vi "Init Log.vi"(8 "error in (no error)":errorcluster, 11 "S4GUI in":refnum<class "S4GUI.lvclass">) -> (0 "error out":errorcluster, 3 "S4GUI out":refnum<class "S4GUI.lvclass">)   [LabVIEW 2018, in "S4GUI.lvclass"]
uses:
  S4GUI.lvclass
  S4GUI.lvclass/S4GUI.ctl
  Log/Log.lvclass
  Acquisition/Acquisition.lvclass
  Instrument/Instrument.lvclass
  TCS/TCS.lvclass
  SyncBox/Sync Box.lvclass
  TelFocus/TelFocus.lvclass
  Comm/Stream/Stream.lvclass
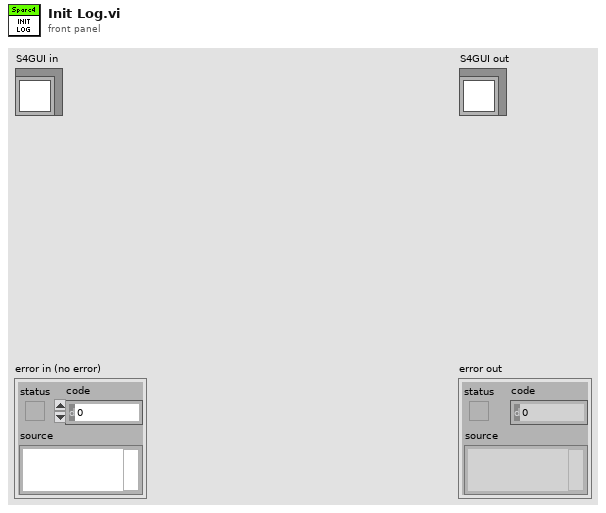
[diagram p1: front panel]
types:
  T1 = enum16{"open", "replace", "create", "open or create", "replace or create", "replace or create with confirmation"}
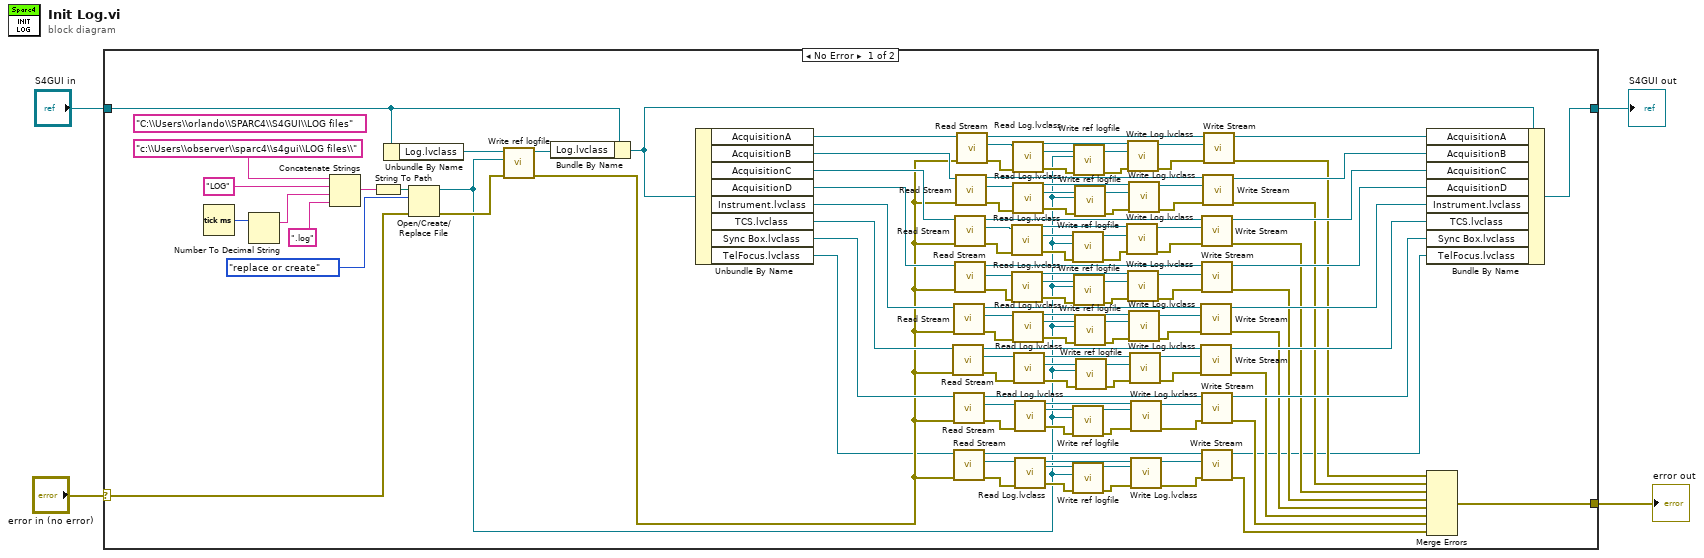
[diagram p0: block diagram]
diagram:
  n1 = case shown="No Error" "error in (no error)" {
    selector: "error in (no error)" -> [w123 w128]
    tunnel: [w98 w128] -> w3
    tunnel: [w120 w127] -> w1
    tunnel: "S4GUI in" -> [w24 w127]
    frame No Error {
      (unwired) "C:\\Users\\orlando\\SPARC4\\S4GUI\\LOG files"
      n2 = Tick Count (ms)() -> (millisecond timer value=w95:u32)
      n3 = Number To Decimal String(number=w95) -> (decimal integer string=w94:string)  [unwired: 1 in]
      n4 = Concatenate Strings("c:\\Users\\observer\\sparc4\\s4gui\\LOG files\\" ("string"), "LOG" ("string"), w94, ".log" ("string")) -> (w124:string)
      n5 = String To Path(string=w124) -> (path=w125:path)
      n6 = Unbundle By Name(w24) -> ("Log.lvclass"=w22:refnum<class "Log.lvclass">)
      n7 = Open/Create/Replace File(file path (use dialog)=w125, error in=w123, operation (0:open)=T1."replace or create") -> (refnum out=w6:refnum<file>, error out=w23:errorcluster)  [unwired: 3 in, 1 out]
      n8 = call-dynamic "Write ref logfile.vi"("error in (no error)"=w23, "ref logfile"=w6, "Log in"=w22) -> ("error out"=w13:errorcluster, "Log out"=w21:refnum<class "Log.lvclass">)  [unwired: 7 in]
      n9 = Bundle By Name(cluster=w24, "Log.lvclass"=w21) -> (w121:refnum<class "S4GUI.lvclass">)
      n10 = Unbundle By Name(w121) -> ("AcquisitionA"=w119:refnum<class "Acquisition.lvclass">, "AcquisitionB"=w118:refnum<class "Acquisition.lvclass">, "AcquisitionC"=w117:refnum<class "Acquisition.lvclass">, "AcquisitionD"=w116:refnum<class "Acquisition.lvclass">, "Instrument.lvclass"=w115:refnum<class "Instrument.lvclass">, "TCS.lvclass"=w114:refnum<class "TCS.lvclass">, "Sync Box.lvclass"=w113:refnum<class "Sync Box.lvclass">, "TelFocus.lvclass"=w12:refnum<class "TelFocus.lvclass">)
      n11 = call-dynamic "Read Stream.vi"("error in (no error)"=w13, "Server in"=w114) -> ("error out"=w30:errorcluster, "Stream.lvclass"=w31:refnum<class "Stream.lvclass">, "Server out"=w34:refnum<class "TCS.lvclass">)  [unwired: 7 in]
      n12 = call-dynamic "Read Stream.vi"("error in (no error)"=w13, "Server in"=w115) -> ("error out"=w46:errorcluster, "Stream.lvclass"=w48:refnum<class "Stream.lvclass">, "Server out"=w49:refnum<class "Instrument.lvclass">)  [unwired: 7 in]
      n13 = call-dynamic "Read Stream.vi"("error in (no error)"=w13, "Server in"=w113) -> ("error out"=w27:errorcluster, "Stream.lvclass"=w28:refnum<class "Stream.lvclass">, "Server out"=w29:refnum<class "Sync Box.lvclass">)  [unwired: 7 in]
      n14 = call-dynamic "Read Stream.vi"("error in (no error)"=w13, "Server in"=w12) -> ("error out"=w15:errorcluster, "Stream.lvclass"=w16:refnum<class "Stream.lvclass">, "Server out"=w11:refnum<class "TelFocus.lvclass">)  [unwired: 7 in]
      n15 = call-dynamic "Read Stream.vi"("error in (no error)"=w13, "Server in"=w117) -> ("error out"=w61:errorcluster, "Stream.lvclass"=w63:refnum<class "Stream.lvclass">, "Server out"=w64:refnum<class "Acquisition.lvclass">)  [unwired: 7 in]
      n16 = call-dynamic "Read Stream.vi"("error in (no error)"=w13, "Server in"=w116) -> ("error out"=w56:errorcluster, "Stream.lvclass"=w55:refnum<class "Stream.lvclass">, "Server out"=w59:refnum<class "Acquisition.lvclass">)  [unwired: 7 in]
      n17 = call-dynamic "Read Stream.vi"("error in (no error)"=w13, "Server in"=w118) -> ("error out"=w79:errorcluster, "Stream.lvclass"=w78:refnum<class "Stream.lvclass">, "Server out"=w76:refnum<class "Acquisition.lvclass">)  [unwired: 7 in]
      n18 = call-dynamic "Read Stream.vi"("error in (no error)"=w13, "Server in"=w119) -> ("error out"=w89:errorcluster, "Stream.lvclass"=w93:refnum<class "Stream.lvclass">, "Server out"=w122:refnum<class "Acquisition.lvclass">)  [unwired: 7 in]
      n19 = call-dynamic "Read Log.lvclass.vi"("error in (no error)"=w61, "Comm in"=w63) -> ("error out"=w71:errorcluster, "Log.lvclass"=w74:refnum<class "Log.lvclass">, "Comm out"=w73:refnum<class "Stream.lvclass">)  [unwired: 7 in]
      n20 = call-dynamic "Read Log.lvclass.vi"("error in (no error)"=w56, "Comm in"=w55) -> ("error out"=w66:errorcluster, "Log.lvclass"=w69:refnum<class "Log.lvclass">, "Comm out"=w68:refnum<class "Stream.lvclass">)  [unwired: 7 in]
      n21 = call-dynamic "Read Log.lvclass.vi"("error in (no error)"=w89, "Comm in"=w93) -> ("error out"=w88:errorcluster, "Log.lvclass"=w92:refnum<class "Log.lvclass">, "Comm out"=w91:refnum<class "Stream.lvclass">)  [unwired: 7 in]
      n22 = call-dynamic "Read Log.lvclass.vi"("error in (no error)"=w79, "Comm in"=w78) -> ("error out"=w81:errorcluster, "Log.lvclass"=w84:refnum<class "Log.lvclass">, "Comm out"=w83:refnum<class "Stream.lvclass">)  [unwired: 7 in]
      n23 = call-dynamic "Read Log.lvclass.vi"("error in (no error)"=w46, "Comm in"=w48) -> ("error out"=w51:errorcluster, "Log.lvclass"=w54:refnum<class "Log.lvclass">, "Comm out"=w53:refnum<class "Stream.lvclass">)  [unwired: 7 in]
      n24 = call-dynamic "Read Log.lvclass.vi"("error in (no error)"=w30, "Comm in"=w31) -> ("error out"=w41:errorcluster, "Log.lvclass"=w44:refnum<class "Log.lvclass">, "Comm out"=w43:refnum<class "Stream.lvclass">)  [unwired: 7 in]
      n25 = call-dynamic "Read Log.lvclass.vi"("error in (no error)"=w27, "Comm in"=w28) -> ("error out"=w36:errorcluster, "Log.lvclass"=w39:refnum<class "Log.lvclass">, "Comm out"=w38:refnum<class "Stream.lvclass">)  [unwired: 7 in]
      n26 = call-dynamic "Read Log.lvclass.vi"("error in (no error)"=w15, "Comm in"=w16) -> ("error out"=w18:errorcluster, "Log.lvclass"=w20:refnum<class "Log.lvclass">, "Comm out"=w9:refnum<class "Stream.lvclass">)  [unwired: 7 in]
      n27 = call-dynamic "Write ref logfile.vi"("error in (no error)"=w71, "ref logfile"=w6, "Log in"=w74) -> ("error out"=w70:errorcluster, "Log out"=w72:refnum<class "Log.lvclass">)  [unwired: 7 in]
      n28 = call-dynamic "Write ref logfile.vi"("error in (no error)"=w36, "ref logfile"=w6, "Log in"=w39) -> ("error out"=w35:errorcluster, "Log out"=w37:refnum<class "Log.lvclass">)  [unwired: 7 in]
      n29 = call-dynamic "Write ref logfile.vi"("error in (no error)"=w18, "ref logfile"=w6, "Log in"=w20) -> ("error out"=w17:errorcluster, "Log out"=w19:refnum<class "Log.lvclass">)  [unwired: 7 in]
      n30 = call-dynamic "Write ref logfile.vi"("error in (no error)"=w88, "ref logfile"=w6, "Log in"=w92) -> ("error out"=w87:errorcluster, "Log out"=w90:refnum<class "Log.lvclass">)  [unwired: 7 in]
      n31 = call-dynamic "Write ref logfile.vi"("error in (no error)"=w66, "ref logfile"=w6, "Log in"=w69) -> ("error out"=w65:errorcluster, "Log out"=w67:refnum<class "Log.lvclass">)  [unwired: 7 in]
      n32 = call-dynamic "Write ref logfile.vi"("error in (no error)"=w81, "ref logfile"=w6, "Log in"=w84) -> ("error out"=w80:errorcluster, "Log out"=w82:refnum<class "Log.lvclass">)  [unwired: 7 in]
      n33 = call-dynamic "Write ref logfile.vi"("error in (no error)"=w51, "ref logfile"=w6, "Log in"=w54) -> ("error out"=w50:errorcluster, "Log out"=w52:refnum<class "Log.lvclass">)  [unwired: 7 in]
      n34 = call-dynamic "Write ref logfile.vi"("error in (no error)"=w41, "ref logfile"=w6, "Log in"=w44) -> ("error out"=w40:errorcluster, "Log out"=w42:refnum<class "Log.lvclass">)  [unwired: 7 in]
      n35 = call-dynamic "Write Log.lvclass.vi"("error in (no error)"=w70, "Log.lvclass"=w72, "Comm in"=w73) -> ("error out"=w60:errorcluster, "Comm out"=w62:refnum<class "Stream.lvclass">)  [unwired: 7 in]
      n36 = call-dynamic "Write Log.lvclass.vi"("error in (no error)"=w87, "Log.lvclass"=w90, "Comm in"=w91) -> ("error out"=w86:errorcluster, "Comm out"=w85:refnum<class "Stream.lvclass">)  [unwired: 7 in]
      n37 = call-dynamic "Write Log.lvclass.vi"("error in (no error)"=w65, "Log.lvclass"=w67, "Comm in"=w68) -> ("error out"=w57:errorcluster, "Comm out"=w58:refnum<class "Stream.lvclass">)  [unwired: 7 in]
      n38 = call-dynamic "Write Log.lvclass.vi"("error in (no error)"=w80, "Log.lvclass"=w82, "Comm in"=w83) -> ("error out"=w75:errorcluster, "Comm out"=w77:refnum<class "Stream.lvclass">)  [unwired: 7 in]
      n39 = call-dynamic "Write Log.lvclass.vi"("error in (no error)"=w50, "Log.lvclass"=w52, "Comm in"=w53) -> ("error out"=w45:errorcluster, "Comm out"=w47:refnum<class "Stream.lvclass">)  [unwired: 7 in]
      n40 = call-dynamic "Write Log.lvclass.vi"("error in (no error)"=w40, "Log.lvclass"=w42, "Comm in"=w43) -> ("error out"=w32:errorcluster, "Comm out"=w33:refnum<class "Stream.lvclass">)  [unwired: 7 in]
      n41 = call-dynamic "Write Log.lvclass.vi"("error in (no error)"=w35, "Log.lvclass"=w37, "Comm in"=w38) -> ("error out"=w26:errorcluster, "Comm out"=w25:refnum<class "Stream.lvclass">)  [unwired: 7 in]
      n42 = call-dynamic "Write Log.lvclass.vi"("error in (no error)"=w17, "Log.lvclass"=w19, "Comm in"=w9) -> ("error out"=w14:errorcluster, "Comm out"=w8:refnum<class "Stream.lvclass">)  [unwired: 7 in]
      n43 = call-dynamic "Write Stream.vi"("error in (no error)"=w45, "Stream.lvclass"=w47, "Server in"=w49) -> ("error out"=w101:errorcluster, "Server out"=w108:refnum<class "Instrument.lvclass">)  [unwired: 7 in]
      n44 = call-dynamic "Write Stream.vi"("error in (no error)"=w32, "Stream.lvclass"=w33, "Server in"=w34) -> ("error out"=w100:errorcluster, "Server out"=w107:refnum<class "TCS.lvclass">)  [unwired: 7 in]
      n45 = call-dynamic "Write Stream.vi"("error in (no error)"=w60, "Stream.lvclass"=w62, "Server in"=w64) -> ("error out"=w103:errorcluster, "Server out"=w110:refnum<class "Acquisition.lvclass">)  [unwired: 7 in]
      n46 = call-dynamic "Write Stream.vi"("error in (no error)"=w57, "Stream.lvclass"=w58, "Server in"=w59) -> ("error out"=w102:errorcluster, "Server out"=w109:refnum<class "Acquisition.lvclass">)  [unwired: 7 in]
      n47 = call-dynamic "Write Stream.vi"("error in (no error)"=w26, "Stream.lvclass"=w25, "Server in"=w29) -> ("error out"=w99:errorcluster, "Server out"=w106:refnum<class "Sync Box.lvclass">)  [unwired: 7 in]
      n48 = call-dynamic "Write Stream.vi"("error in (no error)"=w14, "Stream.lvclass"=w8, "Server in"=w11) -> ("error out"=w7:errorcluster, "Server out"=w10:refnum<class "TelFocus.lvclass">)  [unwired: 7 in]
      n49 = call-dynamic "Write Stream.vi"("error in (no error)"=w75, "Stream.lvclass"=w77, "Server in"=w76) -> ("error out"=w104:errorcluster, "Server out"=w111:refnum<class "Acquisition.lvclass">)  [unwired: 7 in]
      n50 = call-dynamic "Write Stream.vi"("error in (no error)"=w86, "Stream.lvclass"=w85, "Server in"=w122) -> ("error out"=w105:errorcluster, "Server out"=w112:refnum<class "Acquisition.lvclass">)  [unwired: 7 in]
      n51 = Bundle By Name(cluster=w121, "AcquisitionA"=w112, "AcquisitionB"=w111, "AcquisitionC"=w110, "AcquisitionD"=w109, "Instrument.lvclass"=w108, "TCS.lvclass"=w107, "Sync Box.lvclass"=w106, "TelFocus.lvclass"=w10) -> (w120:refnum<class "S4GUI.lvclass">)
      n52 = Merge Errors(w105, w104, w103, w102, w101, w100, w99, w7) -> (w98:errorcluster)
    }
    frame Error {
    }
  }
  "error out" <- w3
  "S4GUI out" <- w1
